vi "Frame2.vi"   [LabVIEW 2014]
uses:
  QwaveSys_Interface/QwaveSys_Interface.lvlib
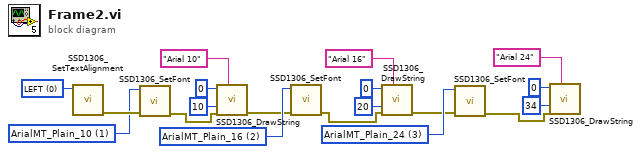
[diagram p0: block diagram]
diagram:
  w8 = u16 3 items=["Crushed_Plain_36", "ArialMT_Plain_10", "ArialMT_Plain_16", "ArialMT_Plain_24"] ("Font")
  w9 = u16 2 items=["Crushed_Plain_36", "ArialMT_Plain_10", "ArialMT_Plain_16", "ArialMT_Plain_24"] ("Font")
  w10 = u16 1 items=["Crushed_Plain_36", "ArialMT_Plain_10", "ArialMT_Plain_16", "ArialMT_Plain_24"] ("Font")
  w11 = u16 0 items=["LEFT", "CENTER", "RIGHT"] ("alignment")
  n1 = call "SSD1306_SetTextAlignment.vi"("alignment"=w11) -> ("error out"=w12:errorcluster)  [unwired: 10 in]
  n2 = call "SSD1306_SetFont.vi"("error in (no error)"=w12, "Font"=w10) -> ("error out"=w7:errorcluster)  [unwired: 9 in]
  n3 = call "SSD1306_DrawString.vi"("String"="Arial 10", "error in (no error)"=w7, "y"=u8 10, "x"=u8 0) -> ("error out"=w6:errorcluster)  [unwired: 7 in]
  n4 = call "SSD1306_SetFont.vi"("error in (no error)"=w6, "Font"=w9) -> ("error out"=w5:errorcluster)  [unwired: 9 in]
  n5 = call "SSD1306_DrawString.vi"("String"="Arial 16", "error in (no error)"=w5, "y"=u8 20, "x"=u8 0) -> ("error out"=w4:errorcluster)  [unwired: 7 in]
  n6 = call "SSD1306_SetFont.vi"("error in (no error)"=w4, "Font"=w8) -> ("error out"=w3:errorcluster)  [unwired: 9 in]
  n7 = call "SSD1306_DrawString.vi"("String"="Arial 24", "error in (no error)"=w3, "y"=u8 34, "x"=u8 0) -> ()  [unwired: 7 in, 1 out]
